vi "Write Min EU.vi"(8 "error in (no error)":errorcluster, 10 "Min EU":dbl, 11 "Frequency in":refnum<class "Frequency.lvclass">) -> (0 "error out":errorcluster, 3 "Frequency out":refnum<class "Frequency.lvclass">)   [LabVIEW 2012, in "Measurement Channels.lvlib" / "Frequency.lvclass"]
uses:
  Frequency.lvclass
  Frequency.lvclass/Frequency.ctl
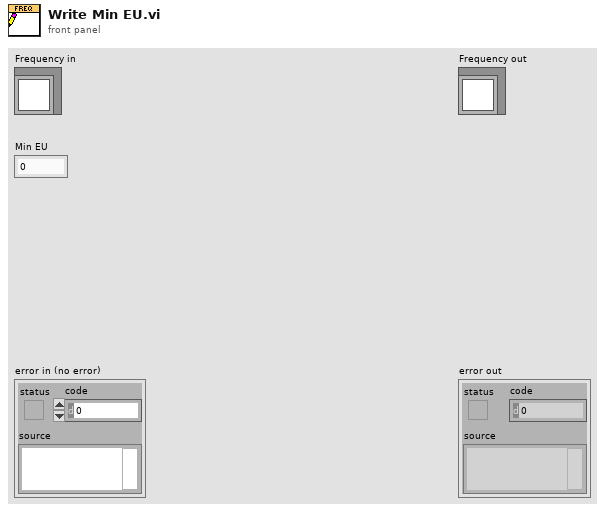
[diagram p1: front panel]
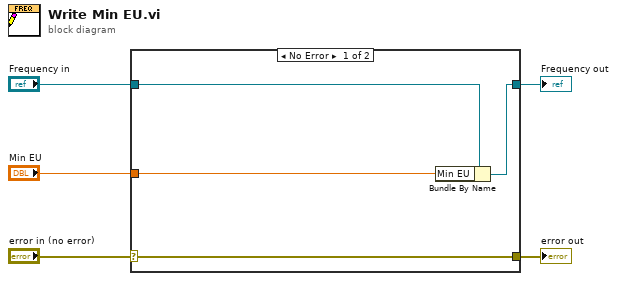
[diagram p0: block diagram]
diagram:
  n1 = case shown="No Error" "error in (no error)" {
    selector: "error in (no error)" -> [w9 w10]
    tunnel: [w9 w10] -> w4
    tunnel: [w7 w11] -> w2
    tunnel: "Frequency in" -> [w8 w11]
    tunnel: "Min EU" -> [w6 _]
    frame No Error {
      n2 = Bundle By Name(cluster=w8, "Min EU"=w6) -> (w7:refnum<class "Frequency.lvclass">)
    }
    frame Error {
    }
  }
  "error out" <- w4
  "Frequency out" <- w2
